vi "oax_Load Data (Digital Tacho).vi"(0 "Data Path In":path, 7 "default relative path":string="Examples\\Order Analysis\\Example Data", 11 "error in (no error)":errorcluster) -> (3 "channel name":string[](array[string]), 4 "vibration data":waveform(dbl)[](array[waveform]), 6 "vibration channel info":T1[](array[typedef]) {"pregain" format="%.2f"; "weighting filter" items=["Linear", "A-weighting", "B-weighting", "C-weighting", "ITU-R 468-4", "Dolby", "CCITT", "C-message", "Wb", "Wc", "Wd", "We", "Wf", "Wh", "Wj", "Wk", "Wm", "AES17 20 kHz lowpass", "AES17 40 kHz lowpass", "AES17 20 kHz highpass", "AES17 40 kHz highpass"]; "dB reference" format="%^.1e"; "engineering units" items=["custom..."=0, "V"=1, "A"=21, "C"=30, "pC"=31, "s"=32, "-"=29, "Pa"=2, "N"=20, "g"=3, "m/s^2"=4, "m/s"=5, "m"=6, "mm/s"=12, "mm"=13, "micron/s"=14, "micron"=15, "in/s^2"=7, "in/s"=8, "in"=9, "mil/s"=10, "mil"=11, "rad/s^2"=16, "rad/s"=17, "rad"=18, "deg/s^2"=26, "deg/s"=27, "deg"=28, "RPM"=22, "cycle/s^2"=23, "Hz"=24, "cycle"=25, "strain"=19]; "sensor sensitivity" format="%#_5f"}, 8 "digital tacho info":T4={"tacho counts"=[], "counter timebase [Hz]"=20000000.0, "counter task type"=enum."event counting", "counter digit (32)"=32}, 14 "pulse / rev":i32, 15 "error out":errorcluster)   [LabVIEW 2017]
doc: "Specify the .ddt file to load vibration and tachometer data from."
uses:
  <vilib>/addons/Sound and Vibration/Order Analysis/Tach Process/SubVIs/digital tach info.ctl
  <vilib>/addons/_NISVFA/_Shared subVIs/Controls/svc_Channel Info.ctl
  <vilib>/addons/_NISVFA/_Shared subVIs/Controls/svc_Engineering Units Text Ring.ctl
  <vilib>/addons/_NISVFA/_Shared subVIs/Controls/svc_Weighting Filter Text Ring.ctl
  <vilib>/addons/Sound and Vibration/Order Analysis/Tach Process/SoundVib_TachProcess.lvlib
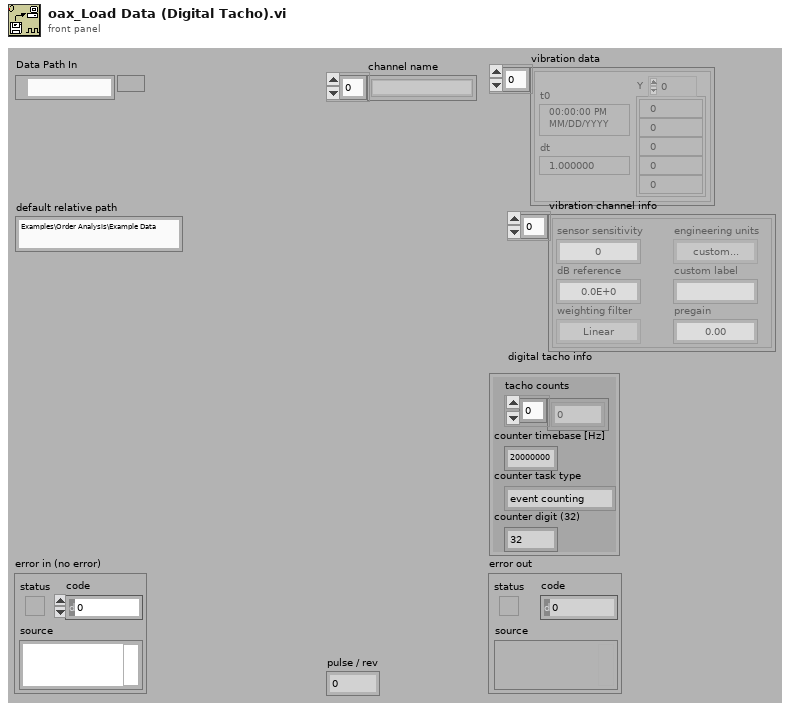
[diagram p1: front panel]
types:
  T1 = typedef "svc_Channel Info.ctl" = cluster{"sensor sensitivity":dbl, "engineering units":T2, "dB reference":dbl, "custom label":string, "weighting filter":T3, "pregain":dbl}
  T2 = typedef "svc_Engineering Units Text Ring.ctl" = u16
  T3 = typedef "svc_Weighting Filter Text Ring.ctl" = u16
  T4 = typedef "SoundVib_TachProcess.lvlib/digital tach info.ctl" = cluster{"tacho counts":i64[], "counter timebase [Hz]":dbl, "counter task type":enum16{"period measurement", "event counting"}, "counter digit (32)":i32}
  T5 = enum16{"open", "open or create", "create or replace", "create", "open (read only)"}
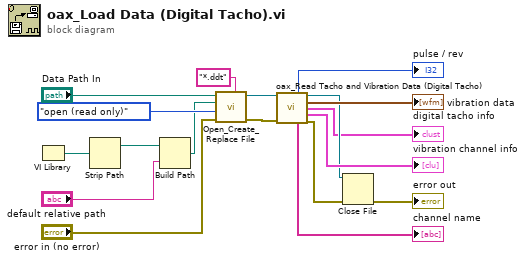
[diagram p0: block diagram]
diagram:
  n1 = VI Library() -> (path=w4:path)
  n2 = Strip Path(path=w4) -> (stripped path=w3:path)  [unwired: 1 out]
  n3 = Build Path(base path=w3, name or relative path="default relative path") -> (appended path=w2:path)
  n4 = call <vilib>:"Open_Create_Replace File.vi"("pattern"="*.ddt", "error in (no error)"="error in (no error)", "function (open:0)"=T5."open (read only)", "start path  (Not A Path)"=w2, "file path"="Data Path In") -> ("error out"=w15:errorcluster, "refnum"=w16:refnum<file>)  [unwired: 3 in, 2 out]
  n5 = call <vilib>:"oax_Read Tacho and Vibration Data (Digital Tacho).vi"("refnum"=w16, "error in (no error)"=w15) -> ("pulse / rev"=→"pulse / rev":i32, "refnum out"=w8:refnum<file>, "waveform data"=→"vibration data":waveform(dbl)[], "digital tacho info"=→"digital tacho info":T4, "channel info"=→"vibration channel info":T1[], "channel name"=→"channel name":string[], "error out"=w7:errorcluster)  [unwired: 7 in]
  n6 = Close File(refnum=w8, error in=w7) -> (error out=→"error out":errorcluster)  [unwired: 1 out]
